vi "stage_home.vi"(8 "error in (no error)":errorcluster, 10 "stage name":string, 11 "newport_xps in":refnum<class "newport_xps.lvclass">) -> (0 "error out":errorcluster, 3 "newport_xps out":refnum<class "newport_xps.lvclass">)   [LabVIEW 2015, in "newport_xps.lvclass"]
uses:
  newport_xps.lvclass
  newport_xps.lvclass/newport_xps.ctl
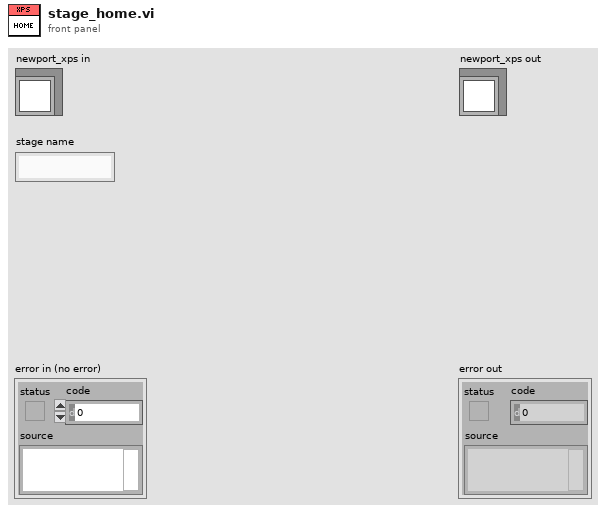
[diagram p1: front panel]
types:
  T1 = cluster{"connection TCP":refnum<k5>, "LogTo File":bool, "Log File refnum":refnum<file>, "no error if error log":bool}
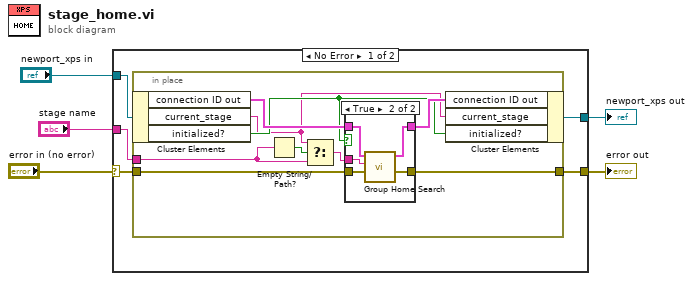
[diagram p0: block diagram]
diagram:
  n1 = case shown="No Error" "error in (no error)" {
    selector: "error in (no error)" -> [w8 w28]
    tunnel: "newport_xps in" -> [w10 w27]
    tunnel: [w9 w27] -> w3
    tunnel: [w7 w28] -> w2
    tunnel: "stage name" -> [w6 _]
    frame No Error {
      n2 = in-place {
        in-place-border: w8 -> [w17]
        in-place-border: [w16] -> w7
        in-place-border: w6 -> [w13]
        n3 = in-place-cluster #1(w10) -> ("connection ID out"=w19:T1, "current_stage"=w11:string, "initialized?"=w15:bool)
        n4 = Empty String/Path?(string/path=w13) -> (empty?=w14:bool)
        n5 = Select(t=w11, s=w14, f=w13) -> (s? t:f=w12:string)
        n6 = case shown="True" w15 {
          tunnel: w19 -> [w20 w26]
          tunnel: [w20 w25] -> w18
          tunnel: w17 -> [w21 w24]
          tunnel: [w21 w23] -> w16
          tunnel: w12 -> [_ w22]
          frame False {
          }
          frame True {
            n7 = call "Group Home Search.vi"("XPS error in (no error)"=w24, "Group Name (250 c max)"=w22, "connection ID in"=w26) -> ("XPS error out"=w23:errorcluster, "connection ID out"=w25:T1)  [unwired: 6 in, 1 out]
          }
        }
        n8 = in-place-cluster #1("connection ID out"=w18, "current_stage"=w11, "initialized?"=w15) -> (w9:refnum<class "newport_xps.lvclass">)
      }
    }
    frame Error {
    }
  }
  "error out" <- w2
  "newport_xps out" <- w3
